vi "Ctx New.vi"(7 "path override":path, 8 "error in (no error)":errorcluster) -> (0 "error out":errorcluster, 3 "function return":u64)   [LabVIEW 2025, in "LibZMQ.lvlib"]
doc: "ZMQ_EXPORT void *zmq_ctx_new (void);"
uses:
  LibZMQ.lvlib
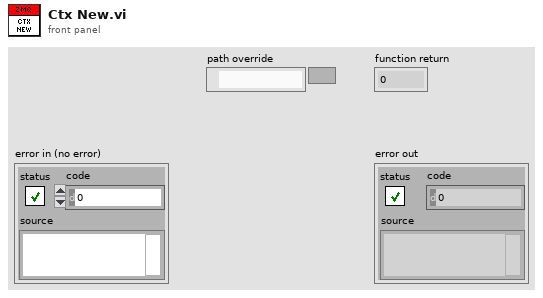
[diagram p1: front panel]
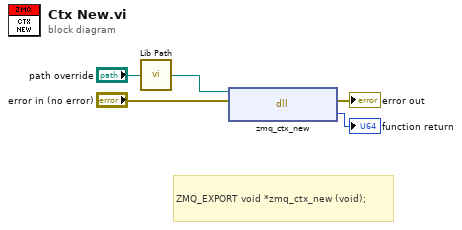
[diagram p0: block diagram]
diagram:
  # "ZMQ_EXPORT void *zmq_ctx_new (void);"
  n1 = call "Lib Path.vi"("path override"="path override") -> ("lib path"=w1:path)
  n2 = dll-call lib="C:/git/ZMQLV/libzmq-v143-mt-4_3_6/lib/win32/libzmq-v143-mt-4_3_6.dll" fn="zmq_ctx_new"(path in=w1, error in="error in (no error)") -> (error out=→"error out":errorcluster, "return type"=→"function return":u64)  [unwired: 1 in, 1 out]
